vi "精简框图4.vi"(0 "P/N:":string, 1 "mid_str_labelType":string="None", 2 "DateCode8Value_0X30":i32, 3 "Convert Style":bool, 4 "LocalDataBase?":bool, 5 "labelConfig":string[](array[string])=["年月日", "16", "16", "17", "17", "", "", "18", "18", "19", "21", "Y050YW(YMD)(S3)"], 6 "mid_array_eep":string[][](array[string])=[["11", "11", "0", "0"], ["7", "0", "0", "0"], ["2", "23", "0", "0"], ["0", "80", "0", "0"], ["0", "0", "0", "0"], ["0", "0", "0", "0"], ["0", "0", "0", "0"], ["0", "0", "0", "0"], ["0", "0", "0", "0"], ["0", "80", "0", "0"], ["0", "0", "0", "0"], ["0", "0", "0", "0"], ["0", "FF", "0", "0"], ["0", "0", "0", "0"], ["0", "0", "0", "0"], ["0", "0", "0", "0"], ["0", "0", "0", "0"], ["0", "0", "0", "0"], ["0", "1", "0", "0"], ["0", "A0", "0", "0"], ["0", "4C", "0", "0"], ["0", "55", "0", "0"], ["0", "58", "0", "0"], ["0", "53", "0", "0"], ["0", "48", "0", "0"], ["0", "41", "0", "0"], ["0", "52", "0", "0"], ["0", "45", "0", "0"], ["0", "2D", "0", "0"], ["0", "49", "0", "0"], ["0", "43", "0", "0"], ["0", "54", "0", "0"], ["0", "20", "0", "0"], ["0", "20", "0", "0"], ["0", "20", "0", "0"], ["0", "20", "0", "0"], ["0", "1F", "0", "0"], ["0", "3C", "0", "0"], ["0", "18", "0", "0"], ["0", "A0", "0", "0"], ["0", "48", "0", "0"], ["0", "48", "0", "0"], ["0", "33", "0", "0"], ["0", "43", "0", "0"], ["0", "30", "0", "0"], ["0", "34", "0", "0"], ["0", "30", "0", "0"], ["0", "34", "0", "0"], ["0", "57", "0", "0"], ["0", "34", "0", "0"], ["0", "31", "0", "0"], ["0", "33", "0", "0"], ["0", "57", "0", "0"], ["0", "58", "0", "0"], ["0", "20", "0", "0"], ["0", "20", "0", "0"], ["0", "41", "0", "0"], ["0", "20", "0", "0"], ["0", "3", "0", "0"], ["0", "4", "0", "0"], ["0", "5", "0", "0"], ["0", "8", "0", "0"], ["0", "46", "0", "0"], ["0", "47", "0", "0"], ["0", "B", "0", "0"], ["0", "0", "0", "0"], ["0", "0", "0", "0"], ["0", "0", "0", "0"], ["0", "31", "0", "0"], ["0", "35", "0", "0"], ["0", "32", "0", "0"], ["0", "32", "0", "0"], ["0", "34", "0", "0"], ["0", "34", "0", "0"], ["0", "30", "0", "0"], ["0", "30", "0", "0"], ["0", "35", "0", "0"], ["0", "20", "0", "0"], ["0", "20", "0", "0"], ["0", "20", "0", "0"], ["0", "20", "0", "0"], ["0", "20", "0", "0"], ["0", "20", "0", "0"], ["0", "20", "0", "0"], ["0", "31", "0", "0"], ["0", "35", "0", "0"], ["0", "30", "0", "0"], ["0", "39", "0", "0"], ["0", "30", "0", "0"], ["0", "31", "0", "0"], ["0", "20", "0", "0"], ["0", "20", "0", "0"], ["0", "0", "0", "0"], ["0", "0", "0", "0"], ["0", "67", "0", "0"], ["0", "89", "0", "0"], ["0", "0", "0", "0"], ["0", "0", "0", "0"], ["0", "0", "0", "0"], ["0", "0", "0", "0"], ["0", "0", "0", "0"], ["0", "0", "0", "0"], ["0", "0", "0", "0"], ["0", "0", "0", "0"], ["0", "0", "0", "0"], ["0", "0", "0", "0"], ["0", "0", "0", "0"], ["0", "0", "0", "0"], ["0", "0", "0", "0"], ["0", "0", "0", "0"], ["0", "0", "0", "0"], ["0", "0", "0", "0"], ["0", "0", "0", "0"], ["0", "0", "0", "0"], ["0", "0", "0", "0"], ["0", "0", "0", "0"], ["0", "0", "0", "0"], ["0", "0", "0", "0"], ["0", "0", "0", "0"], ["0", "0", "0", "0"], ["0", "0", "0", "0"], ["0", "0", "0", "0"], ["0", "0", "0", "0"], ["0", "0", "0", "0"], ["0", "0", "0", "0"], ["0", "0", "0", "0"], ["0", "0", "0", "0"], ["0", "0", "0", "0"]], 7 "SNKeep":bool, 8 "S/N":string="E511D-151101897", 10 "DBSet":T2, 11 "校验信息":T1(array[cluster])) -> (9 "show_date":timestamp, 12 "要烧录的时间和Sn":string, 13 "未经进制转换的sn(客户 jin zhi sn)":string, 14 "要烧录的DateCode":string, 15 "strFSN 原始 Customer sn":string, 16 "输出的label内容":string="CN0T11GF7720661R7005A00#20160127#7005", 17 "Go":bool=TRUE, 20 "mid_array_temp_int":u8[][](array[numeric])=[[3, 4, 33, 0, 0, 0, 0, 65, 4, 128, 213, 0, 103, 0, 0, 0, 0, 0, 0, 0, 0, 0, 0, 0, 0, 0, 0, 0, 0, 0, 0, 0, 0, 0, 0, 0, 0, 0, 0, 0, 0, 0, 0, 0, 0, 0, 0, 0, 0, 0, 0, 0, 0, 0, 0, 0, 0, 0, 0, 0, 1, 0, 0, 42, 0, 0, 0, 0, 0, 0, 0, 0, 0, 0, 0, 0, 0, 0, 0, 0, 0, 0, 0, 0, 49, 52, 49, 49, 50, 53, 0, 0, 0, 0, 0, 46, 0, 0, 0, 0, 0, 0, 0, 0, 0, 0, 0, 0, 0, 0, 0, 0, 0, 0, 0, 0, 0, 0, 0, 0, 0, 0, 0, 0, 0, 0, 0, 0, 0, 0, 0, 0, 0, 0, 0, 0, 0, 0, 0, 0, 0, 0, 0, 0, 0, 0, 0, 0, 0, 0, 0, 0, 0, 0, 0, 0, 0, 0, 0, 0, 0, 0, 0, 0, 0, 0, 0, 0, 0, 0, 0, 0, 0, 0, 0, 0, 0, 0, 0, 0, 0, 0, 0, 0, 0, 0, 0, 0, 0, 0, 0, 0, 0, 0, 0, 0, 0, 0, 0, 0, 0, 0, 0, 0, 0, 0, 0, 0, 0, 0, 0, 0, 0, 0, 0, 0, 0, 0, 0, 0, 0, 0, 0, 0, 0, 0, 0, 0, 0, 0, 0, 0, 0, 0, 0, 0, 0, 0, 0, 0, 0, 0, 0, 0, 0, 0, 0, 0, 0, 0, 0, 0, 0, 0, 0, 0]] format="%.0x", 21 "S/N:":string="153410001", 23 "Customer Date":string, 24 "shi jin zhi sn":string, 25 "Report No.":string="HF-153410001", 27 "Sample #":string="153410001")   [LabVIEW 2011]
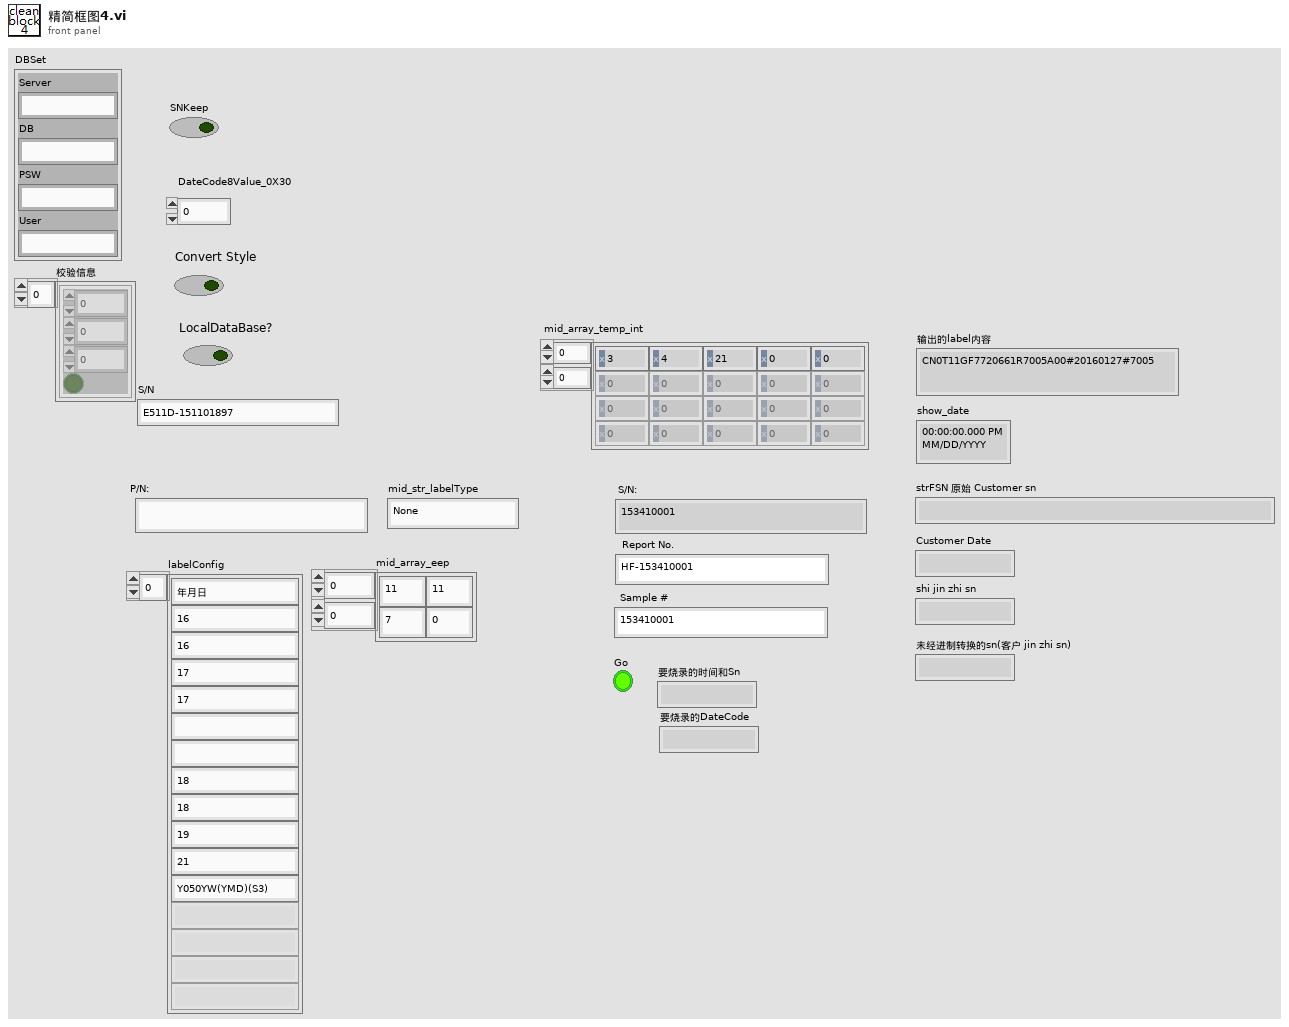
[diagram p1: front panel]
types:
  T1 = cluster{"start":i32, "length":i32, "p":i32, "H/L":bool}[]
  T2 = cluster{"Server":string, "DB":string, "PSW":string, "User":string}
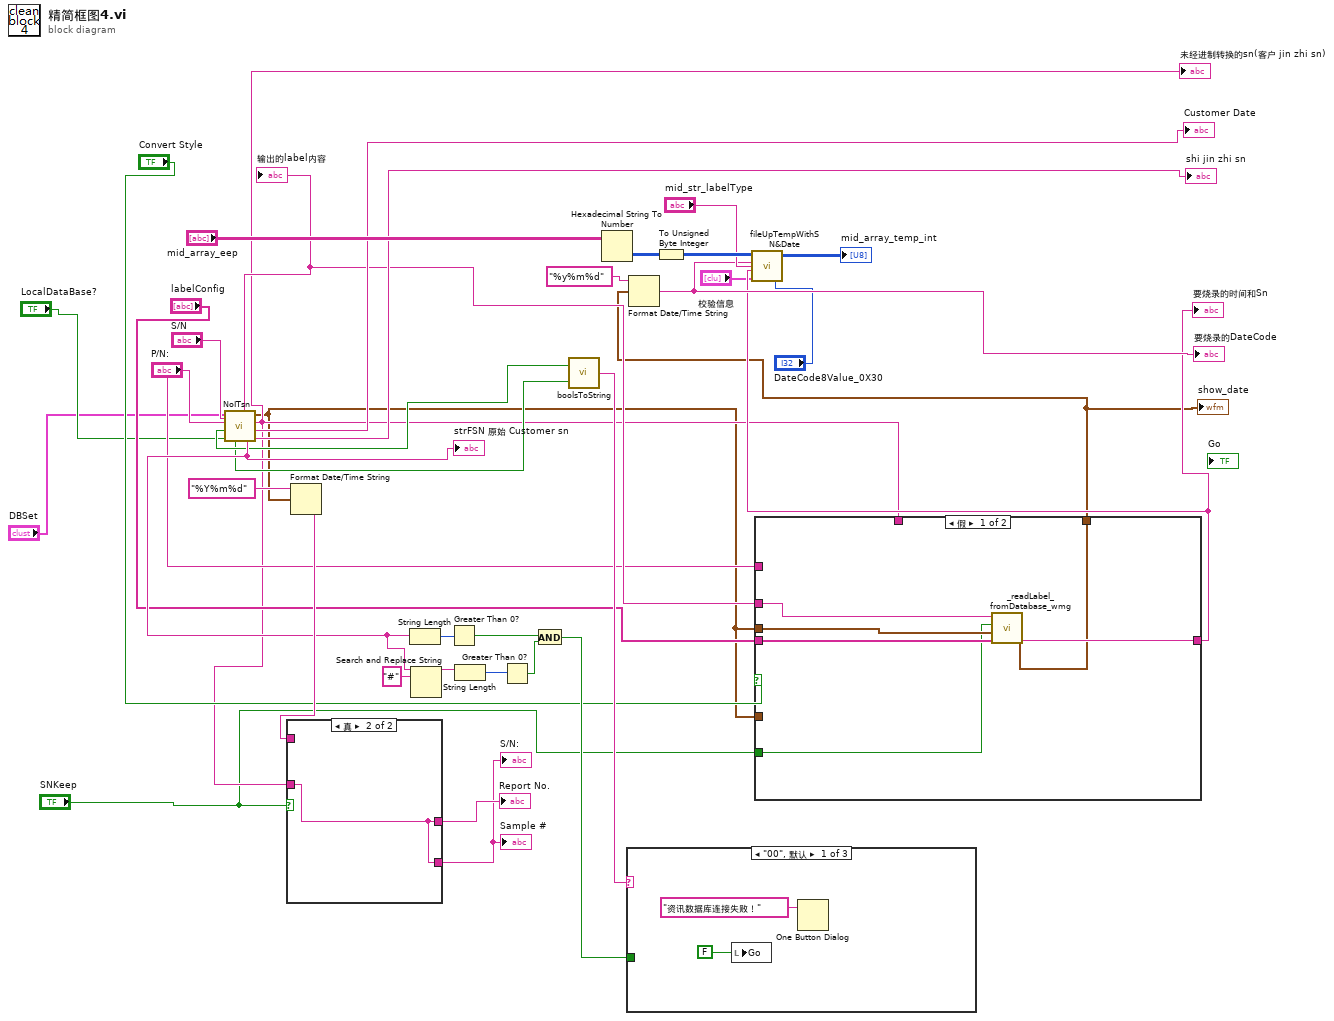
[diagram p0: block diagram]
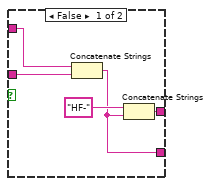
[diagram p2: hidden frame]
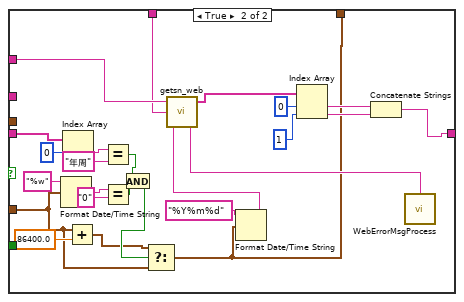
[diagram p3: hidden frame]
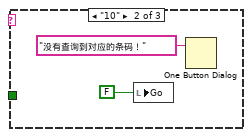
[diagram p4: hidden frame]
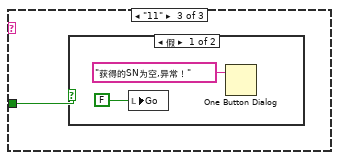
[diagram p5: hidden frame]
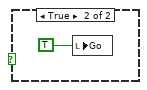
[diagram p6: hidden frame]
diagram:
  n1 = call "NoITsn.vi"("S/N"="S/N", "localDataBase?"="LocalDataBase?", "P/N"="P/N:", "DBSet"="DBSet") -> ("shi jin zhi Sn"=→"shi jin zhi sn":string, "Customer data"=→"Customer Date":string, "未经进制转换的sn(客户 jin zhi sn)"=w8:string, "show_date"=w5:timestamp, "strFSN 原始SN(Include #)"=w16:string, "输出的label内容"=w13:string, "result?"=w14:bool, "status"=w15:bool)
  "输出的label内容" <- w13
  "strFSN 原始 Customer sn" <- w16
  "未经进制转换的sn(客户 jin zhi sn)" <- w8
  n2 = Format Date/Time String(time format string (%c)="%Y%m%d" ("时间格式字符串(%c)"), seconds (now)=w5) -> (date/time string=w33:string)  [unwired: 1 in]
  n3 = case shown="真" "SNKeep" {
    tunnel: w33 -> [w43 _]
    tunnel: [w41 w44] -> w32
    tunnel: [w40 w44] -> w31
    tunnel: w8 -> [w39 w44]
    frame False {
      n4 = Concatenate Strings(w43, w39) -> (w40:string)
      n5 = Concatenate Strings("HF-" ("字符串"), w40) -> (w41:string)
    }
    frame True {
    }
  }
  "S/N:" <- w31
  "Report No." <- w32
  "Sample #" <- w31
  n6 = String Length(string=w16) -> (length=w26:i32)
  n7 = Search and Replace String(input string=w16, search string="#" ("搜索字符串")) -> (result string=w24:string)  [unwired: 6 in, 3 out]
  n8 = Greater Than 0?(x=w26) -> (x > 0?=w22:bool)
  n9 = String Length(string=w24) -> (length=w23:i32)
  n10 = Greater Than 0?(x=w23) -> (x > 0?=w21:bool)
  n11 = And(x=w22, y=w21) -> (x .and. y?=w20:bool)
  n12 = call "boolsToString.vi"("input_bool_low"=w14, "input_bool_high"=w15) -> ("show_str_01string"=w38:string)
  n13 = Hexadecimal String To Number(string="mid_array_eep") -> (number=w37:u32[][])  [unwired: 2 in, 1 out]
  n14 = case shown="\"00\", 默认" w38 {
    tunnel: w20 -> [_ _ w49]
    frame "00", Default {
      n15 = local write "Go"(FALSE ("Go")) -> ()
      n16 = One Button Dialog(message="资讯数据库连接失败！" ("消息")) -> ()  [unwired: 1 in, 1 out]
    }
    frame "10" {
      n17 = local write "Go"(FALSE ("Go")) -> ()
      n18 = One Button Dialog(message="没有查询到对应的条码！" ("消息")) -> ()  [unwired: 1 in, 1 out]
    }
    frame "11" {
      n19 = case shown="假" w49 {
        frame False {
          n20 = local write "Go"(FALSE ("Go")) -> ()
          n21 = One Button Dialog(message="获得的SN为空,异常！" ("消息")) -> ()  [unwired: 1 in, 1 out]
        }
        frame True {
          n22 = local write "Go"(TRUE ("Go")) -> ()
        }
      }
    }
  }
  n23 = To Unsigned Byte Integer(number=w37) -> (unsigned 8bit integer=w35:u8[][])
  n24 = case shown="假" "Convert Style" {
    tunnel: [w58 w77] -> w11
    tunnel: w13 -> [w57 _]
    tunnel: w5 -> [w56 _]
    tunnel: "labelConfig" -> [w55 w74]
    tunnel: w5 -> [_ w61]
    tunnel: "P/N:" -> [_ w76]
    tunnel: w8 -> [_ w75]
    tunnel: [w54 w59] -> w4
    tunnel: "SNKeep" -> [w53 _]
    frame False {
      n25 = call "_readLabel_fromDatabase_wmg.vi"("input_str_label"=w57, "SN keep"=w53, "date"=w56, "input_array_labelConfig"=w55) -> ("show_date"=w54:timestamp, "show_str_snObeyFormat"=w58:string)  [unwired: 3 out]
    }
    frame True {
      n26 = Format Date/Time String(time format string (%c)="%w" ("时间格式字符串(%c)"), seconds (now)=w61) -> (date/time string=w68:string)  [unwired: 1 in]
      n27 = Index Array(array=w74, index=0 ("索引")) -> (element=w72:string)
      n28 = Add(x=w61, y=86400.0) -> (x+y=w62:timestamp)
      n29 = Equal?(x=w72, y="年周") -> (x = y?=w66:bool)
      n30 = Equal?(x=w68, y="0") -> (x = y?=w65:bool)
      n31 = And(x=w66, y=w65) -> (x .and. y?=w64:bool)
      n32 = Select(t=w62, s=w64, f=w61) -> (s? t:f=w59:timestamp)
      n33 = Format Date/Time String(time format string (%c)="%Y%m%d" ("时间格式字符串(%c)"), seconds (now)=w59) -> (date/time string=w60:string)  [unwired: 1 in]
      n34 = call "getsn_web.vi"("strDate"=w60, "sSN"=w75, "strPartNo"=w76) -> ("strErrMsg"=w83:string, "getCode"=w82:string[])  [unwired: 1 out]
      n35 = Index Array(array=w82, index #1=0 ("索引"), index #2=1 ("索引")) -> (element #1=w79:string, element #2=w78:string)
      n36 = Concatenate Strings(w79, w78) -> (w77:string)
      n37 = call "WebErrorMsgProcess.vi"("WebErrorMsg"=w83) -> ()
    }
  }
  "show_date" <- w4
  "要烧录的时间和Sn" <- w11
  n38 = Format Date/Time String(time format string (%c)="%y%m%d" ("时间格式字符串(%c)"), seconds (now)=w4) -> (date/time string=w27:string)  [unwired: 1 in]
  "要烧录的DateCode" <- w27
  n39 = call "fileUpTempWithSN&Date.vi"("input_array_temp_int"=w35, "input_str_Date"=w27, "input_str_SN"=w11, "校验信息"="校验信息", "input_str_customer"="mid_str_labelType", "DateCode8Value_0X30"="DateCode8Value_0X30") -> ("show_array_temp_int"=→"mid_array_temp_int":u8[][])  [unwired: 1 out]
